vi "deleteCmdProj.vi"(1 "num_cmd":string, 2 "Suppression de la commande":bool) -> ()   [LabVIEW 2024]
uses:
  <vilib>/drjdpowell/SQLite Library/SQL Statement/SQL Statement.lvclass/SQL Statement.ctl
  <vilib>/drjdpowell/SQLite Library/SQL Statement/Error Message.vi
  <vilib>/drjdpowell/SQLite Library/SQL Connection/Connection.lvclass
  <vilib>/drjdpowell/SQLite Library/SQLite.lvlib
  <vilib>/drjdpowell/SQLite Library/SQL Connection/Execute SQL.vi
  <vilib>/drjdpowell/SQLite Library/SQL Connection/Open (string).vi
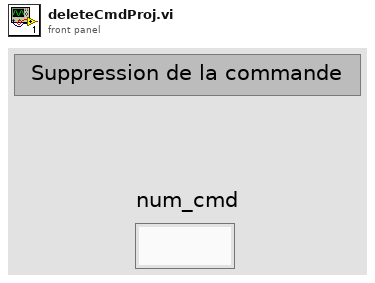
[diagram p1: front panel]
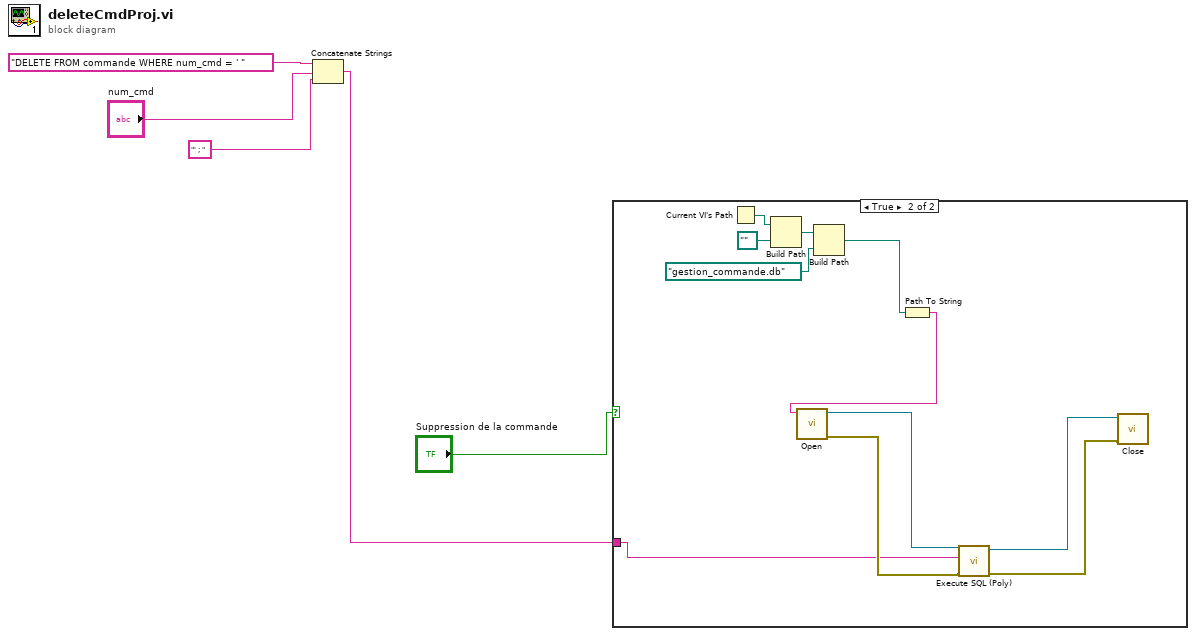
[diagram p0: block diagram]
diagram:
  n1 = Concatenate Strings("DELETE FROM commande WHERE num_cmd = ' " ("SQL"), "num_cmd", "' ; " ("SQL")) -> (w2:string)
  n2 = case shown="True" "Suppression de la commande" {
    tunnel: w2 -> [_ w6]
    frame False {
    }
    frame True {
      n3 = Current VI's Path() -> (path=w16:path)
      n4 = Build Path(base path=w16, name or relative path=path "..") -> (appended path=w13:path)
      n5 = Build Path(base path=w13, name or relative path=path "gestion_commande.db" ("Filename")) -> (appended path=w12:path)
      n6 = Path To String(path=w12) -> (string=w7:string)
      n7 = call-poly <vilib>:"Open.vi"("db file"=w7) -> ("error out"=w11:errorcluster, "SQLite Connection"=w8:refnum<class "Connection.lvclass">)  [unwired: 9 in]
      n8 = call-poly <vilib>:"Execute SQL (Poly).vi"("error in (no error)"=w11, "SQL"=w6, "SQLite Connection in"=w8) -> ("error out"=w10:errorcluster, "SQLite Connection"=w9:refnum<class "Connection.lvclass">)  [unwired: 5 in, 2 out]
      n9 = call-dynamic "Close.vi"("error in (no error)"=w10, "SQLite Connection in"=w9) -> ()  [unwired: 9 in, 1 out]
    }
  }
